vi "Construct Query Component.vi"(10 "HTML Entity (F)":bool, 11 "Query":cluster{"argument":string, "value":string}[](array[cluster])) -> (3 "query":string)   [LabVIEW 2013, in "openURI.lvlib"]
uses:
  openURI.lvlib
  isHEXDigit.vi
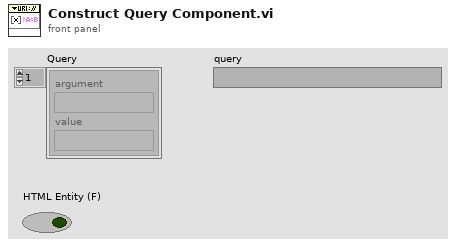
[diagram p1: front panel]
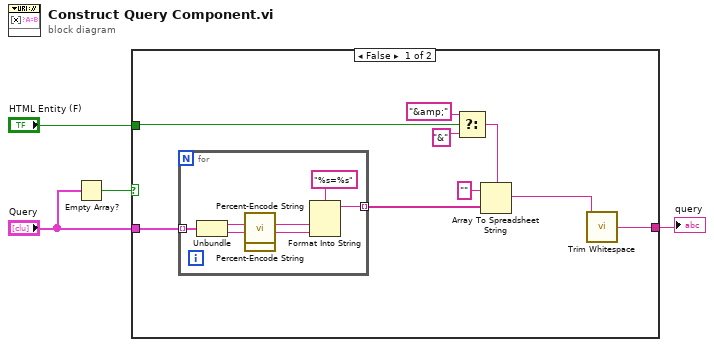
[diagram p0: block diagram]
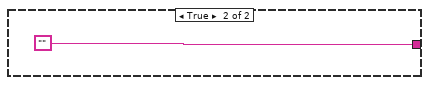
[diagram p2: hidden frame]
diagram:
  n1 = Empty Array?(array="Query") -> (empty?=w4:bool)
  n2 = case shown="False" w4 {
    tunnel: "Query" -> [w13 _]
    tunnel: [w9 ""] -> w2
    tunnel: "HTML Entity (F)" -> [w8 _]
    frame False {
      n3 = for {
        tunnel: w13 -> [w20] mode=indexing
        tunnel: [w18] -> w12 mode=indexing
        n4 = Unbundle(w20) -> ("argument"=w17:string, "value"=w15:string)
        n5 = call "Percent-Encode String.vi"("String"=w17) -> ("Pct-Encoded String"=w16:string)  [unwired: 10 in]
        n6 = call "Percent-Encode String.vi"("String"=w15) -> ("Pct-Encoded String"=w14:string)  [unwired: 10 in]
        n7 = Format Into String(format string="%s=%s", w16, w14) -> (resulting string=w18:string)  [unwired: 2 in, 1 out]
      }
      n8 = Select(t="&amp;" ("delimiter (Tab)"), s=w8, f="&" ("delimiter (Tab)")) -> (s? t:f=w7:string)
      n9 = Array To Spreadsheet String(delimiter (Tab)=w7, array=w12, 3:"" ("format string")) -> (spreadsheet string=w10:string)
      n10 = call <vilib>:"Trim Whitespace.vi"("string"=w10) -> ("trimmed string"=w9:string)  [unwired: 1 in]
    }
    frame True {
    }
  }
  "query" <- w2
